vi "Swerve System (SubVI).vi"(0 "Joystick 1 X (strafe)":dbl(slide) scale=-1.0..1.0, 5 "Joystick 1 Y (forward/back)":dbl(slide) scale=1.0..-1.0, 7 "Joystick 2 X (Rotate)":dbl(slide) scale=-1.0..1.0, 9 "crossLock":bool, 11 "Gyro Angle (deg)":dbl, 12 "moduleAbsoluteAngles":T1) -> (1 "RightFrontWheelPowerDesired":dbl, 2 "LeftFrontWheelPowerDesired":dbl, 3 "LeftRearWheelPowerDesired":dbl, 4 "RightRearWheelPowerDesired":dbl, 6 "rightFrontAngleError":dbl, 8 "leftFrontAngleError":dbl, 10 "leftRearAngleError":dbl, 15 "rightRearAngleError":dbl)   [LabVIEW 2020]
uses:
  TypeDefs/Joysticks.ctl
  Team Code/Robot Global Data.vi
panel:
  in  "Joystick Input":T2
  in  "Trackwidth (W)":dbl=22.5
  in  "Wheelbase (L)":dbl=22.5
  out "invertSpeedRightRear":bool
  out "invertSpeedLeftRear":bool
  out "invertSpeedLeftFront":bool
  out "invertSpeedRightFront":bool
  in  "Hysteresis (deg)":dbl=10.0
  in  "Zero Wheels":bool
  # "Inputs"
  # "Process Variables"
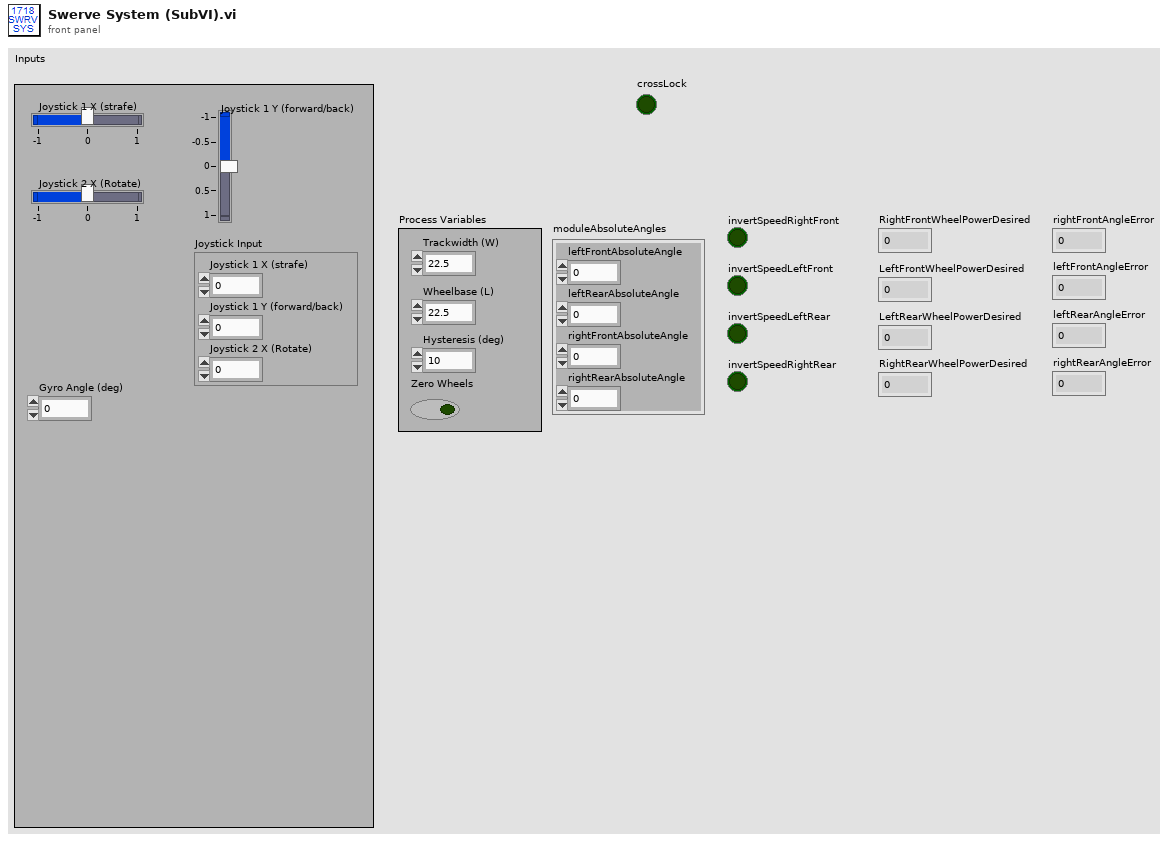
[diagram p1: front panel]
types:
  T1 = cluster{"leftFrontAbsoluteAngle":dbl, "leftRearAbsoluteAngle":dbl, "rightFrontAbsoluteAngle":dbl, "rightRearAbsoluteAngle":dbl}
  T2 = typedef "Joysticks.ctl" = cluster{"Joystick 1 X (strafe)":dbl, "Joystick 1 Y (forward/back)":dbl, "Joystick 2 X (Rotate)":dbl}
  T3 = typedef "WheelPowerDesired.ctl" = cluster{"rightFrontWheelPowerDesired":dbl, "leftFrontWheelPowerDesired":dbl, "leftRearWheelPowerDesired":dbl, "rightRearWheelPowerDesired":dbl}
  T4 = typedef "WheelAngleDesired.ctl" = cluster{"rightFrontWheelAngle":dbl, "leftFrontWheelAngle":dbl, "leftRearWheelAngle":dbl, "rightRearWheelAngle":dbl}
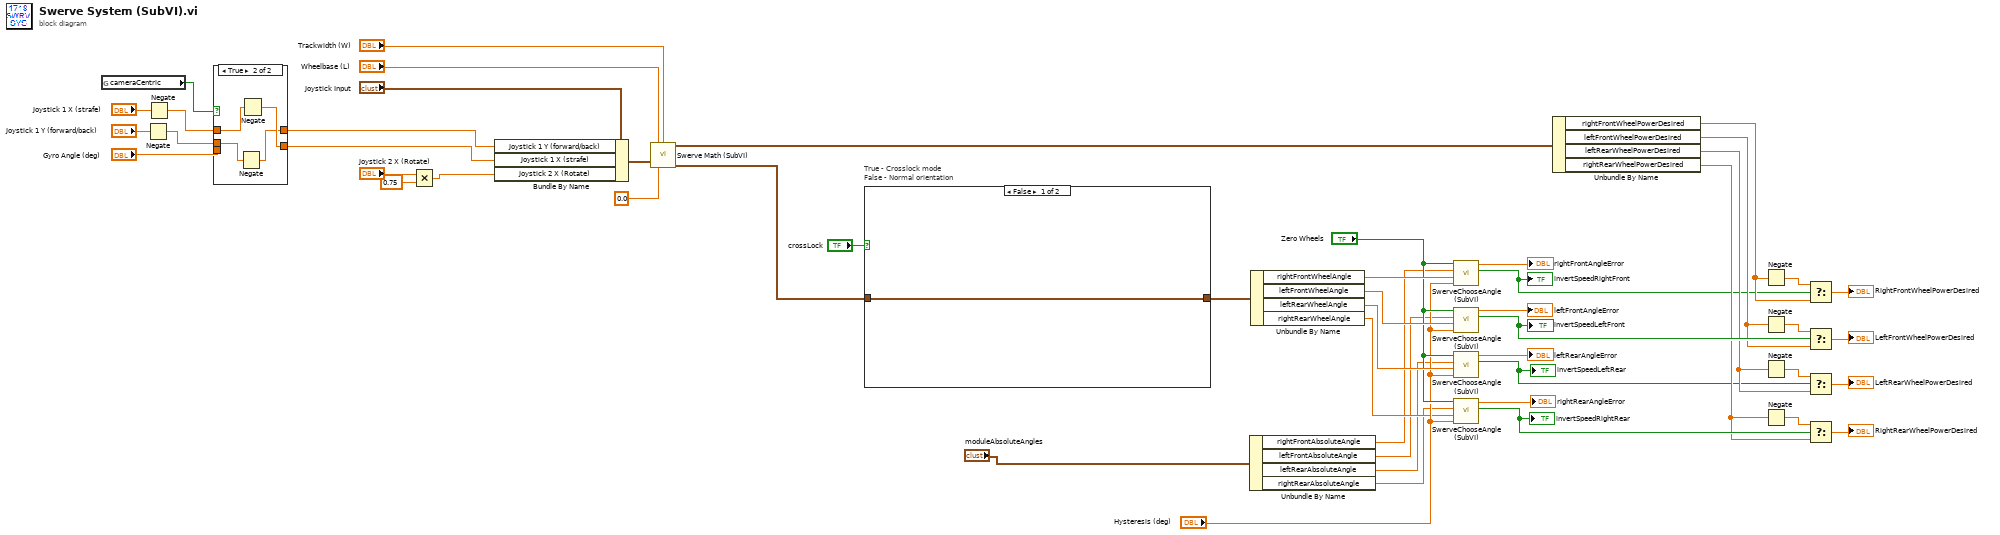
[diagram p0: block diagram]
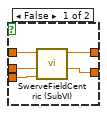
[diagram p2: hidden frame]
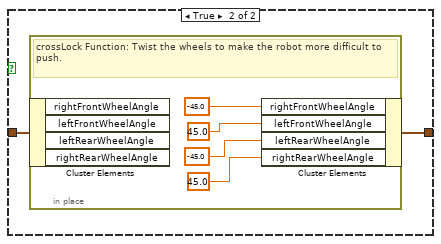
[diagram p3: hidden frame]
diagram:
  n1 = global read "Robot Global Data.vi" "cameraCentric"() -> (w4:bool)
  n2 = Negate(x="Joystick 1 Y (forward/back)") -> (-x=w13:dbl)
  n3 = Negate(x="Joystick 1 X (strafe)") -> (-x=w12:dbl)
  n4 = case shown="True" w4 {
    tunnel: "Gyro Angle (deg)" -> [w56 _]
    tunnel: w13 -> [w55 w58]
    tunnel: w12 -> [w54 w60]
    tunnel: [w53 w57] -> w11
    tunnel: [w52 w59] -> w10
    frame False {
      n5 = call "SwerveFieldCentric (SubVI).vi"("Gyro Angle (deg)"=w56, "Y"=w55, "X"=w54) -> ("X*"=w52:dbl, "Y*"=w53:dbl)  [unwired: 7 in]
    }
    frame True {
      n6 = Negate(x=w58) -> (-x=w57:dbl)
      n7 = Negate(x=w60) -> (-x=w59:dbl)
    }
  }
  n8 = Multiply(x="Joystick 2 X (Rotate)", y=0.75) -> (x*y=w1:dbl)
  n9 = Bundle By Name(cluster="Joystick Input", "Joystick 1 Y (forward/back)"=w11, "Joystick 1 X (strafe)"=w10, "Joystick 2 X (Rotate)"=w1) -> (w48:T2)
  n10 = call "Swerve Math (SubVI).vi"("Wheelbase (L)"="Wheelbase (L)", "Trackwidth (W)"="Trackwidth (W)", "Joystick Input"=w48, "Gyro Angle in degrees"=0.0) -> ("wheelPowerDesired"=w46:T3, "wheelAngleDesired(-180..180)"=w8:T4)  [unwired: 10 in]
  n11 = case "True - Crosslock mode\nFalse - Normal orientation" shown="False" "crossLock" {
    tunnel: w8 -> [w61 w63]
    tunnel: [w61 w62] -> w7
    frame False {
    }
    frame True {
      n12 = in-place {
        # "crossLock Function: Twist the wheels to make the robot more difficult to push."
        n13 = in-place-cluster #1(w63) -> ()  [unwired: 4 out]
        n14 = in-place-cluster #1("rightFrontWheelAngle"=-45.0, "leftFrontWheelAngle"=45.0, "leftRearWheelAngle"=-45.0, "rightRearWheelAngle"=45.0) -> (w62:T4)
      }
    }
  }
  n15 = Unbundle By Name("moduleAbsoluteAngles") -> ("rightFrontAbsoluteAngle"=w22:dbl, "leftFrontAbsoluteAngle"=w21:dbl, "leftRearAbsoluteAngle"=w20:dbl, "rightRearAbsoluteAngle"=w19:dbl)
  n16 = Unbundle By Name(w7) -> ("rightFrontWheelAngle"=w45:dbl, "leftFrontWheelAngle"=w44:dbl, "leftRearWheelAngle"=w43:dbl, "rightRearWheelAngle"=w32:dbl)
  n17 = call "SwerveChooseAngle (SubVI).vi"("Hysteresis (deg)"="Hysteresis (deg)", "Goal Angle (deg)"=w45, "Current Angle (deg)"=w22, "Zero Wheels"="Zero Wheels") -> ("Invert Speed Motor"=w24:bool, "Angular Distance"=→"rightFrontAngleError":dbl)  [unwired: 5 in, 1 out]
  "invertSpeedRightFront" <- w24
  n18 = call "SwerveChooseAngle (SubVI).vi"("Hysteresis (deg)"="Hysteresis (deg)", "Goal Angle (deg)"=w44, "Current Angle (deg)"=w21, "Zero Wheels"="Zero Wheels") -> ("Invert Speed Motor"=w34:bool, "Angular Distance"=→"leftFrontAngleError":dbl)  [unwired: 5 in, 1 out]
  "invertSpeedLeftFront" <- w34
  n19 = call "SwerveChooseAngle (SubVI).vi"("Hysteresis (deg)"="Hysteresis (deg)", "Goal Angle (deg)"=w43, "Current Angle (deg)"=w20, "Zero Wheels"="Zero Wheels") -> ("Invert Speed Motor"=w27:bool, "Angular Distance"=→"leftRearAngleError":dbl)  [unwired: 5 in, 1 out]
  "invertSpeedLeftRear" <- w27
  n20 = call "SwerveChooseAngle (SubVI).vi"("Hysteresis (deg)"="Hysteresis (deg)", "Goal Angle (deg)"=w32, "Current Angle (deg)"=w19, "Zero Wheels"="Zero Wheels") -> ("Invert Speed Motor"=w33:bool, "Angular Distance"=→"rightRearAngleError":dbl)  [unwired: 5 in, 1 out]
  "invertSpeedRightRear" <- w33
  n21 = Unbundle By Name(w46) -> ("rightFrontWheelPowerDesired"=w31:dbl, "leftFrontWheelPowerDesired"=w30:dbl, "leftRearWheelPowerDesired"=w29:dbl, "rightRearWheelPowerDesired"=w28:dbl)
  n22 = Negate(x=w31) -> (-x=w50:dbl)
  n23 = Negate(x=w30) -> (-x=w39:dbl)
  n24 = Negate(x=w29) -> (-x=w38:dbl)
  n25 = Negate(x=w28) -> (-x=w35:dbl)
  n26 = Select(t=w50, s=w24, f=w31) -> (s? t:f=→"RightFrontWheelPowerDesired":dbl)
  n27 = Select(t=w39, s=w34, f=w30) -> (s? t:f=→"LeftFrontWheelPowerDesired":dbl)
  n28 = Select(t=w38, s=w27, f=w29) -> (s? t:f=→"LeftRearWheelPowerDesired":dbl)
  n29 = Select(t=w35, s=w33, f=w28) -> (s? t:f=→"RightRearWheelPowerDesired":dbl)
